vi "MDML_send_config.vi"(8 "error in (no error)":errorcluster, 9 "connMeta 3":T1, 10 "Experiment ID":string, 11 "Configuration filepath":path) -> (0 "error out":errorcluster)   [LabVIEW 2018]
uses:
  Downloads/mqtt_lv2013_201708181938/mqtt_lv2013/mqtt Folder/src/class/mqtt/mqttTypedef/mqttConnectionMeta.ctl
  Downloads/mqtt_lv2013_201708181938/mqtt_lv2013/mqtt Folder/src/class/mqtt/mqttTypedef/mqttQOSlevel.ctl
  Downloads/mqtt_lv2013_201708181938/mqtt_lv2013/mqtt Folder/src/class/mqtt/mqtt.lvclass
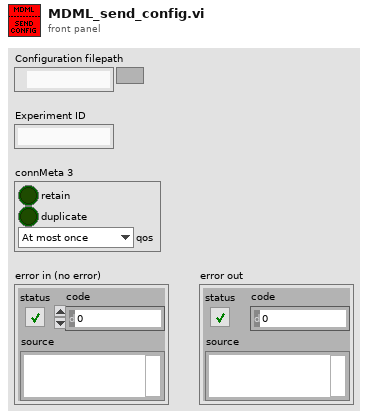
[diagram p1: front panel]
types:
  T1 = typedef "mqttConnectionMeta.ctl" = cluster{"retain":bool, "duplicate":bool, "qos":T2}
  T2 = typedef "mqttQOSlevel.ctl" = enum8{"At most once", "At least once", "Exactly once", "Reserved"}
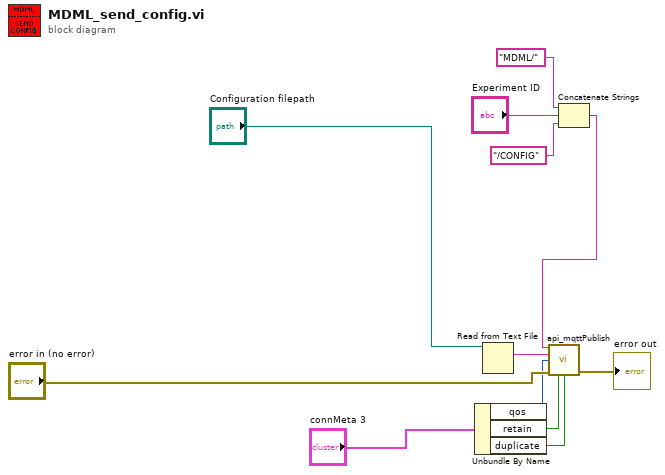
[diagram p0: block diagram]
diagram:
  n1 = Unbundle By Name("connMeta 3") -> ("qos"=w8:T2, "retain"=w9:bool, "duplicate"=w10:bool)
  n2 = Read from Text File(file (use dialog)="Configuration filepath") -> (text=w6:string)  [unwired: 3 in, 3 out]
  n3 = Concatenate Strings("MDML/", "Experiment ID", "/CONFIG") -> (w1:string)
  n4 = call "api_mqttPublish.vi"("topic"=w1, "value"=w6, "QoS (At most once)"=w8, "error in (no error)"="error in (no error)", "retain(F)"=w9, "duplicate(F)"=w10) -> ("error out"=→"error out":errorcluster)  [unwired: 8 in, 1 out]
